vi "Set function value frequnecy AR.vi"(4 "Function (F0 - V DC)":T1(ring), 6 "Voltage frequnecy limit (none)":T2(ring), 7 "Ignore intr. errors (false)":bool, 8 "error in":errorcluster, 9 "Frequency [Hz]":dbl=10.0 min=10.0 max=1000000.0, 10 "Value":dbl, 11 "VISA resource name":refnum<visa-resource-name>) -> (0 "error out":errorcluster, 2 "Setup failed":bool, 3 "VISA resource name out":refnum<visa-resource-name>)   [LabVIEW 2020, in "Datron D4xxx.lvlib"]
doc: "Sets function using \"Set function\" and value and frequency using \"Set value and frequency\" VI. Options are the same as in theese VIs."
uses:
  Datron D4xxx.lvlib
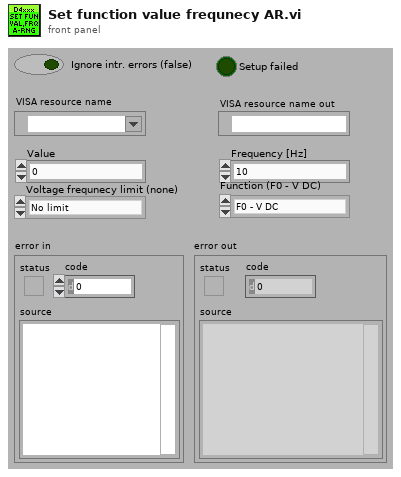
[diagram p1: front panel]
types:
  T1 = enum16{"F0 - V DC", "F1 - V AC", "F2 - A DC", "F3 - A AC", "F4 - R", "F5 - V WB"}
  T2 = enum16{"No limit", "Always to 1kHz", "D4800", "D4805", "D4808"}
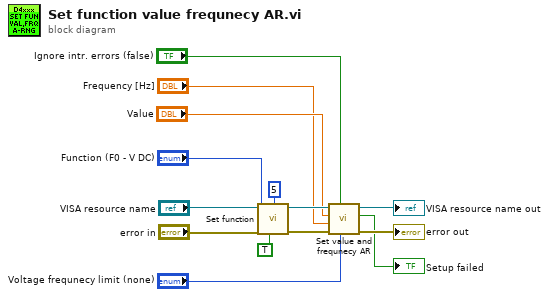
[diagram p0: block diagram]
diagram:
  n1 = call "Set function.vi"("Allow reset (false)"=TRUE, "error in"="error in", "Initial range (R5)"=5, "Function (F0 - V DC)"="Function (F0 - V DC)", "VISA resource name"="VISA resource name") -> ("error out"=w11:errorcluster, "VISA resource name out"=w12:refnum<visa-resource-name>)  [unwired: 5 in]
  n2 = call "Set value and frequnecy AR.vi"("Voltage frequnecy limit (none)"="Voltage frequnecy limit (none)", "Ignore intr. errors (false)"="Ignore intr. errors (false)", "error in"=w11, "Frequency [Hz]"="Frequency [Hz]", "Value"="Value", "VISA resource name"=w12) -> ("error out"=→"error out":errorcluster, "Setup failed"=→"Setup failed":bool, "VISA resource name out"=→"VISA resource name out":refnum<visa-resource-name>)  [unwired: 3 in]
